vi "Finish.vi"(4 "error in":errorcluster) -> ()   [LabVIEW 2013]
doc: "This VI is called just before exiting. It is expected to close I/O refnum, save collected data, etc."
uses:
  <vilib>/Rock Robotics/WPI/Solenoid/WPI_SolenoidValue.ctl
  <vilib>/Rock Robotics/WPI/Compressor/WPI_CompressorGetSetRefNum.vi
  <vilib>/Rock Robotics/WPI/RobotDrive/WPI_RobotDriveGetSetRefNum.vi
  <vilib>/Rock Robotics/WPI/Joystick/WPI_JoystickGetSetRefNum.vi
  <vilib>/Rock Robotics/WPI/Solenoid/WPI_SolenoidSetEnum.vi
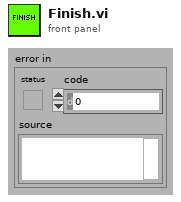
[diagram p1: front panel]
types:
  T1 = typedef "WPI_DigitalInputDevRef.ctl" = cluster{"DevStatus":errorcluster, "DIO Channel":T2, "Digital Module":T3}
  T2 = typedef "FPGA_DIOChannel.ctl" = enum8{"DIO 1", "DIO 2", "DIO 3", "DIO 4", "DIO 5", "DIO 6", "DIO 7", "DIO 8", "DIO 9", "DIO 10", "DIO 11", "DIO 12", "DIO 13", "DIO 14", "Invalid"}
  T3 = typedef "FPGA_TypedefDigitalModule.ctl" = enum16{"Digital Module 1", "Digital Module 2"}
  T4 = typedef "WPI_JoystickDevRef.ctl" = cluster{"Device":T5}
  T5 = typedef "WPI_JoystickDeviceEnum.ctl" = enum16{"USB 1", "USB 2", "USB 3", "USB 4", "Kinect 1", "Kinect 2"}
  T6 = typedef "WPI_CameraDevRef.ctl" = cluster{"Camera Address":string, "CameraStatus":errorcluster, "Acquire Image Notifier":refnum<notifier>}
  T7 = typedef "WPI_RobotDriveDevRef.ctl" = cluster{"DevStatus":errorcluster, "Motors[]":T8[], "Square Inputs":bool, "Max Output":dbl, "Isochronous":bool}
  T8 = typedef "WPI_MotorControlDeviceRef.ctl" = cluster{"DeviceStatus":errorcluster, "Type":enum16{"PWM", "CAN"}, "PWM":cluster{"Digital Module":T3, "PWM Channel":T9, "DeadBand":T10}, "CAN":cluster{"Device Number":u8, "Control Mode":T11, "Semaphore":T12, "Max Vout":dbl}, "Invert":bool, "TransformRef":T13, "InvTransformRef":T13}
  T9 = typedef "FPGA_DIOPWMChannel.ctl" = enum8{"PWM 1", "PWM 2", "PWM 3", "PWM 4", "PWM 5", "PWM 6", "PWM 7", "PWM 8", "PWM 9", "PWM 10", "Invalid"}
  T10 = typedef "WPI_PWMDeadband.ctl" = cluster{"Name":string, "maxPositivePwm":i32, "minPositivePwm":i32, "centerPwm":i32, "maxNegativePwm":i32, "minNegativePwm":i32, "angularRange":u16}
  T11 = typedef "WPI_CANJaguar_ControlMode.ctl" = enum8{"Percent VBus", "Current", "Speed", "Position", "Voltage"}
  T12 = typedef "Semaphore RefNum" = refnum<k1>
  T13 = typedef "WPI_PWMTransform_ConPane.ctl" = refnum<vi>
  T14 = typedef "WPI_EncoderDevRef.ctl" = cluster{"DevStatus":errorcluster, "EncoderIndex":T15, "CounterIndex":T16, "DistancePerCount":dbl, "Decoding Type":T17}
  T15 = typedef "FPGA_EncoderIdx.ctl" = enum8{"Enc 0", "Enc 1", "Enc 2", "Enc 3", "Invalid"}
  T16 = typedef "FPGA_CounterCtrSystemIndex.ctl" = enum8{"Ctr 0", "Ctr 1", "Ctr 2", "Ctr 3", "Ctr 4", "Ctr 5", "Ctr 6", "Ctr 7", "Invalid"}
  T17 = typedef "WPI_EncoderType.ctl" = enum16{"1x", "2x", "4x"}
  T18 = typedef "WPI_SolenoidDevRef.ctl" = cluster{"DevStatus":errorcluster, "Solenoid Module":T19, "Forward Solenoid Channel":T20, "Reverse Solenoid Channel":T20}
  T19 = typedef "FPGA_TypedefSolenoidModule.ctl" = enum16{"Solenoid Module 1", "Solenoid Module 2"}
  T20 = typedef "WPI_SolenoidChannel.ctl" = enum8{"Solenoid 1", "Solenoid 2", "Solenoid 3", "Solenoid 4", "Solenoid 5", "Solenoid 6", "Solenoid 7", "Solenoid 8", "Invalid"}
  T21 = typedef "WPI_CompressorDevRef.ctl" = cluster{"DevStatus":errorcluster, "DigitalInputDevRef":T1, "RelayDevRef":T22}
  T22 = typedef "WPI_RelayDevRef.ctl" = cluster{"DevStatus":errorcluster, "Relay Channel":T23, "Digital Module":T3, "Relay Direction":T24}
  T23 = typedef "FPGA_DIORelayChannel.ctl" = enum8{"Relay 1", "Relay 2", "Relay 3", "Relay 4", "Relay 5", "Relay 6", "Relay 7", "Relay 8", "Invalid"}
  T24 = typedef "WPI_RelayDirection.ctl" = enum16{"Both directions", "Forward only", "Reverse only"}
  T25 = typedef "WPI_SolenoidValue.ctl" = enum16{"Off", "On", "Forward", "Reverse"}
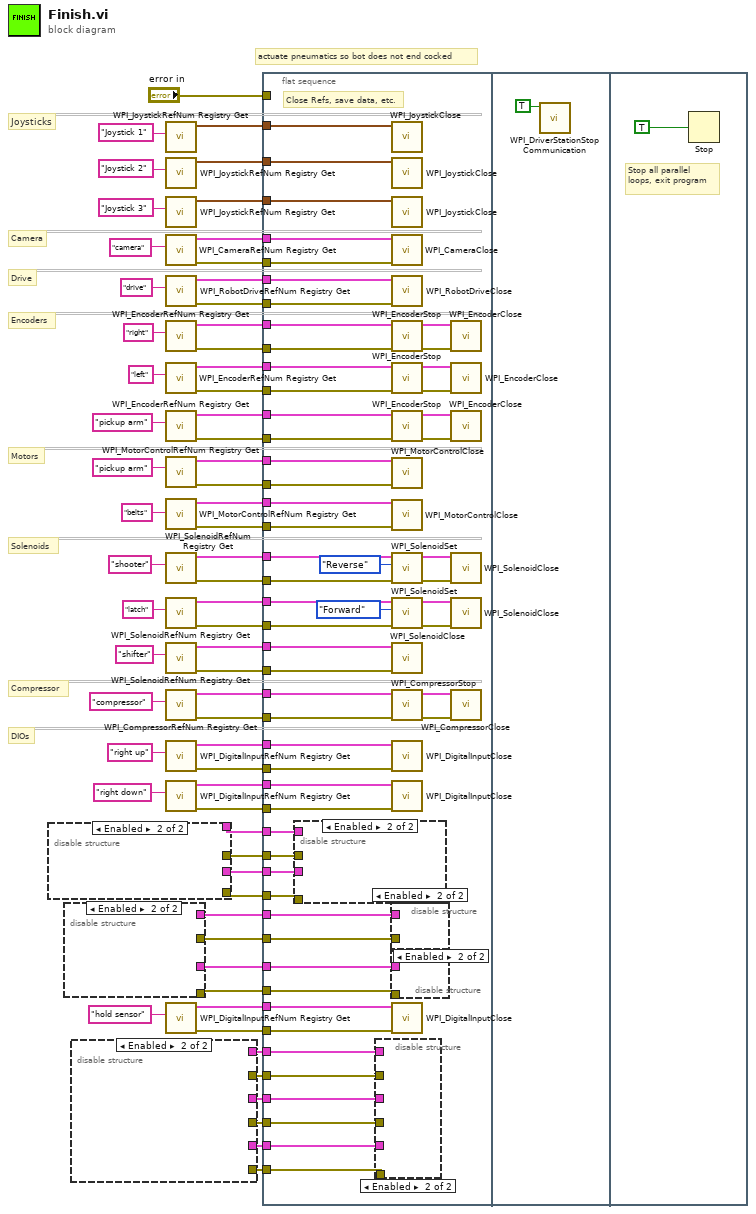
[diagram p0: block diagram]
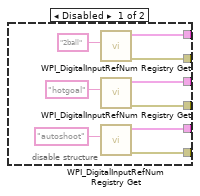
[diagram p2: hidden frame]
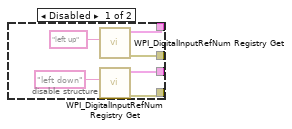
[diagram p3: hidden frame]
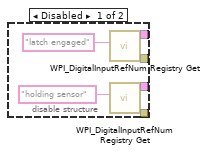
[diagram p4: hidden frame]
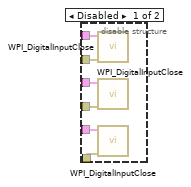
[diagram p5: hidden frame]
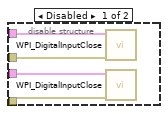
[diagram p6: hidden frame]
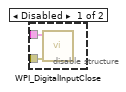
[diagram p7: hidden frame]
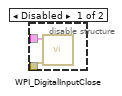
[diagram p8: hidden frame]
diagram:
  # "Compressor"
  # "Joysticks"
  # "Camera"
  # "Drive"
  # "Encoders"
  # "Motors"
  # "Solenoids"
  # "DIOs"
  # "actuate pneumatics so bot does not end cocked"
  n1 = disable-structure shown="Enabled" {
    disable-tunnel: [w67 _] -> w23
    disable-tunnel: [w66 _] -> w22
    disable-tunnel: [w65 _] -> w21
    disable-tunnel: [w64 _] -> w20
    frame Disabled {
      n2 = call <vilib>:"WPI_DigitalInputRefNum Registry Get.vi"("refnum name"="left up") -> ("error out"=w66:errorcluster, "DigitalInputDevRef"=w67:T1)  [unwired: 9 in]
      n3 = call <vilib>:"WPI_DigitalInputRefNum Registry Get.vi"("refnum name"="left down") -> ("error out"=w64:errorcluster, "DigitalInputDevRef"=w65:T1)  [unwired: 9 in]
    }
    frame Enabled {
    }
  }
  n4 = disable-structure shown="Enabled" {
    disable-tunnel: [w75 _] -> w17
    disable-tunnel: [w74 _] -> w16
    disable-tunnel: [w72 _] -> w14
    disable-tunnel: [w71 _] -> w13
    frame Disabled {
      n5 = call <vilib>:"WPI_DigitalInputRefNum Registry Get.vi"("refnum name"="latch engaged") -> ("error out"=w72:errorcluster, "DigitalInputDevRef"=w71:T1)  [unwired: 9 in]
      n6 = call <vilib>:"WPI_DigitalInputRefNum Registry Get.vi"("refnum name"="holding sensor") -> ("error out"=w75:errorcluster, "DigitalInputDevRef"=w74:T1)  [unwired: 9 in]
    }
    frame Enabled {
    }
  }
  n7 = disable-structure shown="Enabled" {
    disable-tunnel: [w84 _] -> w12
    disable-tunnel: [w83 _] -> w11
    disable-tunnel: [w81 _] -> w10
    disable-tunnel: [w80 _] -> w9
    disable-tunnel: [w79 _] -> w8
    disable-tunnel: [w78 _] -> w7
    frame Disabled {
      n8 = call <vilib>:"WPI_DigitalInputRefNum Registry Get.vi"("refnum name"="2ball") -> ("error out"=w83:errorcluster, "DigitalInputDevRef"=w84:T1)  [unwired: 9 in]
      n9 = call <vilib>:"WPI_DigitalInputRefNum Registry Get.vi"("refnum name"="hotgoal") -> ("error out"=w81:errorcluster, "DigitalInputDevRef"=w80:T1)  [unwired: 9 in]
      n10 = call <vilib>:"WPI_DigitalInputRefNum Registry Get.vi"("refnum name"="autoshoot") -> ("error out"=w78:errorcluster, "DigitalInputDevRef"=w79:T1)  [unwired: 9 in]
    }
    frame Enabled {
    }
  }
  n11 = call <vilib>:"WPI_JoystickRefNum Registry Get.vi"("refnum name"="Joystick 1") -> ("JoystickDevRef"=w62:T4)  [unwired: 1 in, 9 out]
  n12 = call <vilib>:"WPI_JoystickRefNum Registry Get.vi"("refnum name"="Joystick 2") -> ("JoystickDevRef"=w59:T4)  [unwired: 1 in, 9 out]
  n13 = call <vilib>:"WPI_JoystickRefNum Registry Get.vi"("refnum name"="Joystick 3") -> ("JoystickDevRef"=w56:T4)  [unwired: 1 in, 9 out]
  n14 = call <vilib>:"WPI_CameraRefNum Registry Get.vi"("refnum name"="camera") -> ("error out"=w49:errorcluster, "CameraDevRef"=w61:T6)  [unwired: 1 in, 8 out]
  n15 = call <vilib>:"WPI_RobotDriveRefNum Registry Get.vi"("refnum name"="drive") -> ("error out"=w48:errorcluster, "RobotDriveDevRef"=w54:T7)  [unwired: 9 in]
  n16 = call <vilib>:"WPI_EncoderRefNum Registry Get.vi"("refnum name"="right") -> ("error out"=w47:errorcluster, "EncoderDevRef"=w51:T14)  [unwired: 9 in]
  n17 = call <vilib>:"WPI_EncoderRefNum Registry Get.vi"("refnum name"="left") -> ("error out"=w46:errorcluster, "EncoderDevRef"=w50:T14)  [unwired: 9 in]
  n18 = call <vilib>:"WPI_EncoderRefNum Registry Get.vi"("refnum name"="pickup arm") -> ("error out"=w45:errorcluster, "EncoderDevRef"=w43:T14)  [unwired: 9 in]
  n19 = call <vilib>:"WPI_MotorControlRefNum Registry Get.vi"("refnum name"="pickup arm") -> ("error out"=w39:errorcluster, "MotorControlDevRef"=w40:T8)  [unwired: 9 in]
  n20 = call <vilib>:"WPI_MotorControlRefNum Registry Get.vi"("refnum name"="belts") -> ("error out"=w37:errorcluster, "MotorControlDevRef"=w38:T8)  [unwired: 9 in]
  n21 = call <vilib>:"WPI_SolenoidRefNum Registry Get.vi"("refnum name"="shooter") -> ("error out"=w35:errorcluster, "SolenoidDevRef"=w36:T18)  [unwired: 9 in]
  n22 = call <vilib>:"WPI_SolenoidRefNum Registry Get.vi"("refnum name"="latch") -> ("error out"=w31:errorcluster, "SolenoidDevRef"=w32:T18)  [unwired: 9 in]
  n23 = call <vilib>:"WPI_SolenoidRefNum Registry Get.vi"("refnum name"="shifter") -> ("error out"=w5:errorcluster, "SolenoidDevRef"=w6:T18)  [unwired: 9 in]
  n24 = call <vilib>:"WPI_CompressorRefNum Registry Get.vi"("refnum name"="compressor") -> ("error out"=w1:errorcluster, "CompressorDevRef"=w2:T21)  [unwired: 9 in]
  n25 = call <vilib>:"WPI_DigitalInputRefNum Registry Get.vi"("refnum name"="right up") -> ("error out"=w26:errorcluster, "DigitalInputDevRef"=w27:T1)  [unwired: 9 in]
  n26 = call <vilib>:"WPI_DigitalInputRefNum Registry Get.vi"("refnum name"="right down") -> ("error out"=w24:errorcluster, "DigitalInputDevRef"=w25:T1)  [unwired: 9 in]
  n27 = call <vilib>:"WPI_DigitalInputRefNum Registry Get.vi"("refnum name"="hold sensor") -> ("error out"=w19:errorcluster, "DigitalInputDevRef"=w18:T1)  [unwired: 9 in]
  n28 = flat-sequence {
    tunnel: w62 -> [w143]
    tunnel: w61 -> [w142]
    tunnel: w59 -> [w141]
    tunnel: w56 -> [w140]
    tunnel: w54 -> [w139]
    tunnel: w51 -> [w138]
    tunnel: w50 -> [w131]
    tunnel: w49 -> [w135]
    tunnel: w48 -> [w134]
    tunnel: w47 -> [w133]
    tunnel: w46 -> [w132]
    tunnel: w45 -> [w127]
    tunnel: w43 -> [w126]
    tunnel: w40 -> [w124]
    tunnel: w39 -> [w123]
    tunnel: w38 -> [w121]
    tunnel: w37 -> [w122]
    tunnel: w36 -> [w104]
    tunnel: w35 -> [w103]
    tunnel: w32 -> [w100]
    tunnel: w31 -> [w99]
    tunnel: "error in" -> [_]
    tunnel: w27 -> [w116]
    tunnel: w26 -> [w117]
    tunnel: w25 -> [w115]
    tunnel: w24 -> [w118]
    tunnel: w23 -> [w114]
    tunnel: w22 -> [w119]
    tunnel: w21 -> [w113]
    tunnel: w20 -> [w120]
    tunnel: w16 -> [w111]
    tunnel: w17 -> [w110]
    tunnel: w18 -> [w112]
    tunnel: w19 -> [w109]
    tunnel: w13 -> [w108]
    tunnel: w14 -> [w107]
    tunnel: w12 -> [w105]
    tunnel: w11 -> [w106]
    tunnel: w9 -> [w94]
    tunnel: w10 -> [w93]
    tunnel: w8 -> [w91]
    tunnel: w7 -> [w92]
    tunnel: w6 -> [w90]
    tunnel: w5 -> [w89]
    tunnel: w2 -> [w88]
    tunnel: w1 -> [w87]
    frame #0 {
      # "Close Refs, save data, etc."
      n29 = disable-structure shown="Enabled" {
        disable-tunnel: w120 -> [w153 _]
        disable-tunnel: w119 -> [w152 _]
        disable-tunnel: w114 -> [w151 _]
        disable-tunnel: w113 -> [w150 _]
        frame Disabled {
          n30 = call <vilib>:"WPI_DigitalInputClose.vi"("error in (no error)"=w152, "DigitalInputDevRef"=w151) -> ()  [unwired: 9 in, 1 out]
          n31 = call <vilib>:"WPI_DigitalInputClose.vi"("error in (no error)"=w153, "DigitalInputDevRef"=w150) -> ()  [unwired: 9 in, 1 out]
        }
        frame Enabled {
        }
      }
      n32 = disable-structure shown="Enabled" {
        disable-tunnel: w106 -> [w149 _]
        disable-tunnel: w105 -> [w148 _]
        disable-tunnel: w94 -> [w147 _]
        disable-tunnel: w93 -> [w146 _]
        disable-tunnel: w92 -> [w145 _]
        disable-tunnel: w91 -> [w144 _]
        frame Disabled {
          n33 = call <vilib>:"WPI_DigitalInputClose.vi"("error in (no error)"=w149, "DigitalInputDevRef"=w148) -> ()  [unwired: 9 in, 1 out]
          n34 = call <vilib>:"WPI_DigitalInputClose.vi"("error in (no error)"=w146, "DigitalInputDevRef"=w147) -> ()  [unwired: 9 in, 1 out]
          n35 = call <vilib>:"WPI_DigitalInputClose.vi"("error in (no error)"=w145, "DigitalInputDevRef"=w144) -> ()  [unwired: 9 in, 1 out]
        }
        frame Enabled {
        }
      }
      n36 = call <vilib>:"WPI_JoystickClose.vi"("JoystickDevRef"=w143) -> ()  [unwired: 11 out]
      n37 = call <vilib>:"WPI_JoystickClose.vi"("JoystickDevRef"=w141) -> ()  [unwired: 11 out]
      n38 = call <vilib>:"WPI_JoystickClose.vi"("JoystickDevRef"=w140) -> ()  [unwired: 11 out]
      n39 = call <vilib>:"WPI_CameraClose.vi"("error in (no error)"=w135, "CameraDevRef"=w142) -> ()  [unwired: 10 out]
      n40 = call <vilib>:"WPI_RobotDriveClose.vi"("error in (no error)"=w134, "RobotDriveDevRef"=w139) -> ()  [unwired: 9 in, 1 out]
      n41 = call <vilib>:"WPI_EncoderStop.vi"("error in (no error)"=w133, "EncoderDevRef"=w138) -> ("error out"=w137:errorcluster, "EncoderDevRef"=w136:T14)  [unwired: 8 in]
      n42 = call <vilib>:"WPI_EncoderStop.vi"("error in (no error)"=w132, "EncoderDevRef"=w131) -> ("error out"=w129:errorcluster, "EncoderDevRef"=w130:T14)  [unwired: 8 in]
      n43 = call <vilib>:"WPI_EncoderStop.vi"("error in (no error)"=w127, "EncoderDevRef"=w126) -> ("error out"=w128:errorcluster, "EncoderDevRef"=w125:T14)  [unwired: 8 in]
      n44 = call <vilib>:"WPI_MotorControlClose.vi"("error in (no error)"=w123, "MotorControlDevRef"=w124) -> ()  [unwired: 9 in, 1 out]
      n45 = call <vilib>:"WPI_MotorControlClose.vi"("error in (no error)"=w122, "MotorControlDevRef"=w121) -> ()  [unwired: 9 in, 1 out]
      n46 = call-poly <vilib>:"WPI_SolenoidSet.vi"("error in (no error)"=w103, "Value"=WPI_SolenoidValue."Reverse", "SolenoidDevRef"=w104) -> ("error out"=w96:errorcluster, "SolenoidDevRef"=w95:T18)  [unwired: 7 in]
      n47 = call-poly <vilib>:"WPI_SolenoidSet.vi"("error in (no error)"=w99, "Value"=WPI_SolenoidValue."Forward", "SolenoidDevRef"=w100) -> ("error out"=w102:errorcluster, "SolenoidDevRef"=w101:T18)  [unwired: 7 in]
      n48 = call <vilib>:"WPI_SolenoidClose.vi"("error in (no error)"=w89, "SolenoidDevRef"=w90) -> ()  [unwired: 9 in, 1 out]
      n49 = call <vilib>:"WPI_CompressorStop.vi"("error in (no error)"=w87, "CompressorDevRef"=w88) -> ("error out"=w86:errorcluster, "CompressorDevRef"=w85:T21)  [unwired: 8 in]
      n50 = call <vilib>:"WPI_DigitalInputClose.vi"("error in (no error)"=w117, "DigitalInputDevRef"=w116) -> ()  [unwired: 9 in, 1 out]
      n51 = call <vilib>:"WPI_DigitalInputClose.vi"("error in (no error)"=w118, "DigitalInputDevRef"=w115) -> ()  [unwired: 9 in, 1 out]
      n52 = disable-structure shown="Enabled" {
        disable-tunnel: w108 -> [w155 _]
        disable-tunnel: w107 -> [w154 _]
        frame Disabled {
          n53 = call <vilib>:"WPI_DigitalInputClose.vi"("error in (no error)"=w154, "DigitalInputDevRef"=w155) -> ()  [unwired: 9 in, 1 out]
        }
        frame Enabled {
        }
      }
      n54 = disable-structure shown="Enabled" {
        disable-tunnel: w111 -> [w157 _]
        disable-tunnel: w110 -> [w156 _]
        frame Disabled {
          n55 = call <vilib>:"WPI_DigitalInputClose.vi"("error in (no error)"=w156, "DigitalInputDevRef"=w157) -> ()  [unwired: 9 in, 1 out]
        }
        frame Enabled {
        }
      }
      n56 = call <vilib>:"WPI_DigitalInputClose.vi"("error in (no error)"=w109, "DigitalInputDevRef"=w112) -> ()  [unwired: 9 in, 1 out]
      n57 = call <vilib>:"WPI_EncoderClose.vi"("error in (no error)"=w137, "EncoderDevRef"=w136) -> ()  [unwired: 9 in, 1 out]
      n58 = call <vilib>:"WPI_EncoderClose.vi"("error in (no error)"=w129, "EncoderDevRef"=w130) -> ()  [unwired: 9 in, 1 out]
      n59 = call <vilib>:"WPI_EncoderClose.vi"("error in (no error)"=w128, "EncoderDevRef"=w125) -> ()  [unwired: 9 in, 1 out]
      n60 = call <vilib>:"WPI_SolenoidClose.vi"("error in (no error)"=w96, "SolenoidDevRef"=w95) -> ()  [unwired: 9 in, 1 out]
      n61 = call <vilib>:"WPI_SolenoidClose.vi"("error in (no error)"=w102, "SolenoidDevRef"=w101) -> ()  [unwired: 9 in, 1 out]
      n62 = call <vilib>:"WPI_CompressorClose.vi"("error in (no error)"=w86, "CompressorDevRef"=w85) -> ()  [unwired: 9 in, 1 out]
    }
    frame #1 {
      n63 = call <vilib>:"WPI_DriverStationStop Communication.vi"("StopCommunication"=TRUE) -> ()  [unwired: 10 in, 1 out]
    }
    frame #2 {
      # "Stop all parallel\nloops, exit program"
      n64 = Stop(stop? (T)=TRUE ("Quit")) -> ()
    }
  }
